vi "Filename_ouput.vi"(3 "Error in (no error)":errorcluster, 5 "Application ref in":refnum<vi>) -> (0 "error out":errorcluster, 1 "Next filename":path caption="filename", 2 "Application ref out":refnum<vi>)   [LabVIEW 2025]
uses:
  <userlib>/Nanonis Prog Interface V5/Nanonis Prog Interface.lvlib
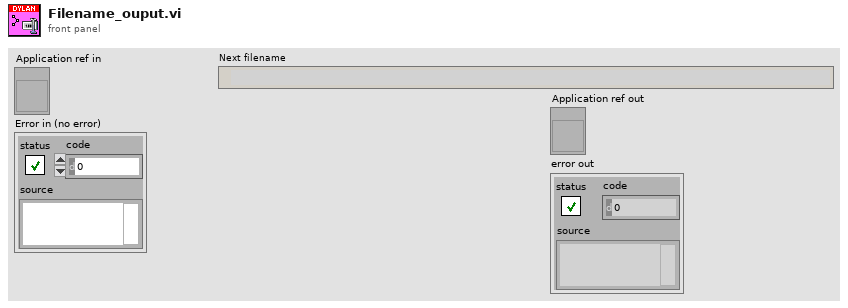
[diagram p1: front panel]
types:
  T1 = cluster{"Path":path, "Basename":string, "Extension":string}
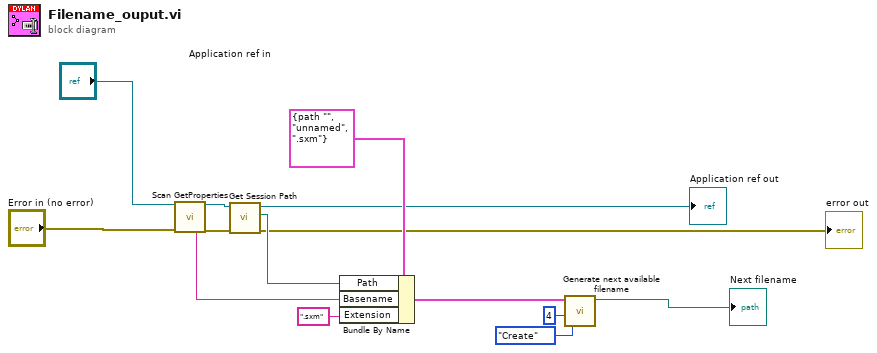
[diagram p0: block diagram]
diagram:
  n1 = call <userlib>:"Scan GetProperties.vi"("Application ref in"="Application ref in", "Error in (no error)"="Error in (no error)") -> ("Application ref out"=w14:refnum<vi>, "Serie name"=w11:string, "Error out"=w13:errorcluster)  [unwired: 6 in, 5 out]
  n2 = call <userlib>:"Get Session Path.vi"("error in (no error)"=w13, "Application ref in"=w14) -> ("error out"=→"error out":errorcluster, "Session path"=w12:path, "Application ref out"=→"Application ref out":refnum<vi>)  [unwired: 7 in]
  n3 = Bundle By Name(cluster=T1 {"Path"=path "", "Basename"="unnamed", "Extension"=".sxm"} ("Filename control"), "Path"=w12, "Basename"=w11, "Extension"=".sxm") -> (w9:T1)
  n4 = call <userlib>:"Generate next available filename.vi"("Mode (Create)"=enum16{"Preview", "Create"}."Create", "Number of digits (3)"=u8 4, "Filename control"=w9) -> ("Next filename"=→"Next filename":path)  [unwired: 3 in, 1 out]
